vi "VariantInit.vi"(3 "Container State":T5, 4 "Previous State":variant, 5 "Previous Version":T4) -> (2 "Current State":T1)   [LabVIEW 2011, in "VariantXControl__VP.xctl"]
uses:
  VariantXControl__VP.xctl
  VariantState.ctl
  Permissions.ctl
  TreeSettings.ctl
  <vilib>/_xctls/Container State.ctl
  <vilib>/_xctls/Version.ctl
  <vilib>/_xctls/XControlSupport.lvlib
panel:
  in  "Default Indicator State":T1={"State"="", "Messages"=[], "Current run"=0, "Start run"=0, "LastTag"="", "Tags"=[], "Length"=0, "Permissions"={"Reset"=TRUE, "TraverseAttributes"=TRUE, "Colorize"=TRUE}, "IsProbe?"=FALSE, "Changed"=FALSE, "TreeSettings"={"Traverse"=TRUE, "Colorize"=TRUE}, "Tree Ref"=refnum}
  in  "Default Control State":T1={"State"="", "Messages"=[], "Current run"=0, "Start run"=0, "LastTag"="", "Tags"=[], "Length"=0, "Permissions"={"Reset"=TRUE, "TraverseAttributes"=TRUE, "Colorize"=TRUE}, "IsProbe?"=FALSE, "Changed"=FALSE, "TreeSettings"={"Traverse"=TRUE, "Colorize"=TRUE}, "Tree Ref"=refnum}
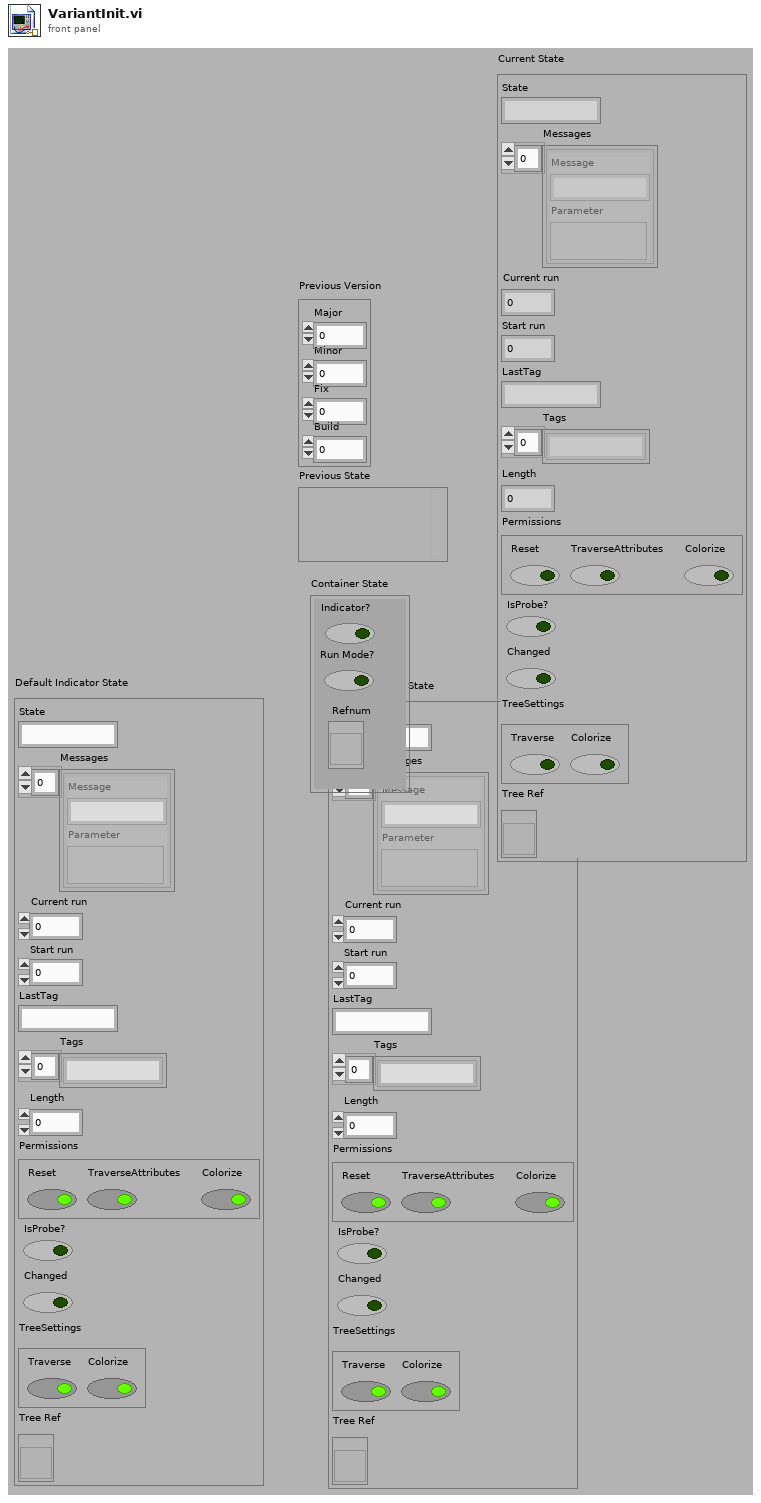
[diagram p1: front panel]
types:
  T1 = typedef "VariantXControl__VP.xctl/VariantState.ctl" = cluster{"State":string, "Messages":cluster{"Message":string, "Parameter":variant}[], "Current run":i32, "Start run":i32, "LastTag":string, "Tags":string[], "Length":i32, "Permissions":T2, "IsProbe?":bool, "Changed":bool, "TreeSettings":T3, "Tree Ref":refnum<vi>}
  T2 = typedef "VariantXControl__VP.xctl/Permissions.ctl" = cluster{"Reset":bool, "TraverseAttributes":bool, "Colorize":bool}
  T3 = typedef "VariantXControl__VP.xctl/TreeSettings.ctl" = cluster{"Traverse":bool, "Colorize":bool}
  T4 = typedef "XControlSupport.lvlib/Version.ctl" = cluster{"Major":u16, "Minor":u16, "Fix":u16, "Build":u16}
  T5 = typedef "XControlSupport.lvlib/Container State.ctl" = cluster{"Indicator?":bool, "Run Mode?":bool, " Refnum":refnum<vi>}
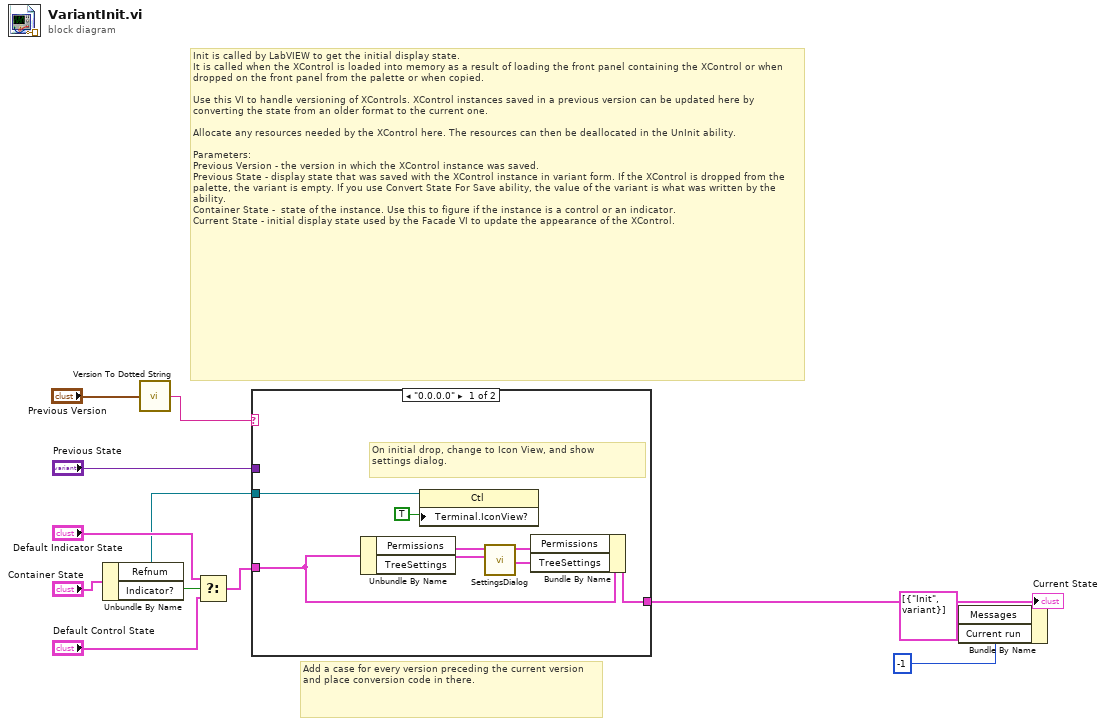
[diagram p0: block diagram]
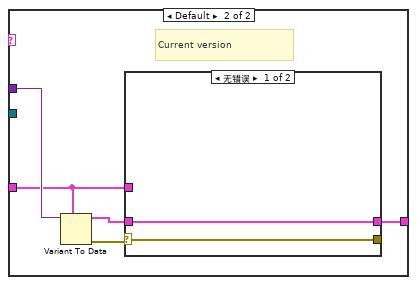
[diagram p2: hidden frame]
diagram:
  # "Add a case for every version preceding the current version and place conversion code in there."
  # "Init is called by LabVIEW to get the initial display state.\nIt is called when the XControl is loaded into memory as a result of loading the front panel containing the XControl or when dropped on the front panel from the palette or when copied.\n\nUse this VI to handle versioning of XControls. XControl instances saved in a previous version can be updated here by converting the state from an older format to the current one.\n\nAllocate any resources needed by the XControl here. The resources can then be deallocated in the UnInit ability.\n\nParameters:\nPrevious Version - the version in which the XControl instance was saved.\nPrevious State - display state that was saved with the XControl instance in variant form. If the XControl is dropped from the palette, the variant is empty. If you use Convert State For Save ability, the value of the variant is what was written by the ability. \nContainer State -  state of the instance. Use this to figure if the instance is a control or an indicator.\nCurrent State - initial display state used by the Facade VI to update the appearance of the XControl."
  n1 = Unbundle By Name("Container State") -> ("Refnum"=w1:refnum<vi>, "Indicator?"=w9:bool)
  n2 = call <vilib>:"Version To Dotted String.vi"("Version"="Previous Version") -> ("String Version"=w10:string)
  n3 = Select(t="Default Indicator State", s=w9, f="Default Control State") -> (s? t:f=w6:T1)
  n4 = case shown="\"0.0.0.0\"" w10 {
    tunnel: "Previous State" -> [_ w26]
    tunnel: [w16 w22] -> w3
    tunnel: w6 -> [w19 w23]
    tunnel: w1 -> [w20 _]
    frame "0.0.0.0" {
      # "On initial drop, change to Icon View, and show\nsettings dialog."
      n5 = Unbundle By Name(w19) -> ("Permissions"=w18:T2, "TreeSettings"=w17:T3)
      n6 = property class="Ctl"(reference=w20, "Terminal.IconView?"=TRUE ("Terminal.Icon View?")) -> ()  [unwired: 1 in, 2 out]
      n7 = call "SettingsDialog.vi"("TreeSettings In"=w17, "Settings In"=w18) -> ("TreeSettings Out"=w14:T3, "Settings Out"=w15:T2)  [unwired: 8 in]
      n8 = Bundle By Name(cluster=w19, "Permissions"=w15, "TreeSettings"=w14) -> (w16:T1)
    }
    frame Default {
      # "Current version"
      n9 = Variant To Data(type=w23, Variant=w26) -> (data=w24:T1, error out=w25:errorcluster)  [unwired: 1 in]
      n10 = case shown="无错误" w25 {
        selector: w25 -> [w28 w29]
        tunnel: w24 -> [w27 _]
        tunnel: [w27 w30] -> w22
        tunnel: w23 -> [_ w30]
        tunnel: [w28 w29] -> _
        frame No Error {
        }
        frame Error {
          # "Error converting previously \nsaved state. Use default instead."
        }
      }
    }
  }
  n11 = Bundle By Name(cluster=w3, "Messages"=cluster{"Message":string, "Parameter":variant}[] [{"Message"="Init", "Parameter"=variant}], "Current run"=-1) -> (→"Current State":T1)
